vi "Get Points.vi"(11 "Task Base in":refnum<class "Task Base.lvclass">) -> (2 "Points":string[](array[string]), 3 "Task Base out":refnum<class "Task Base.lvclass">)   [LabVIEW 2023, in "Task Base.lvclass"]
uses:
  Task Base.lvclass
  Task Base.lvclass/Task Base.ctl
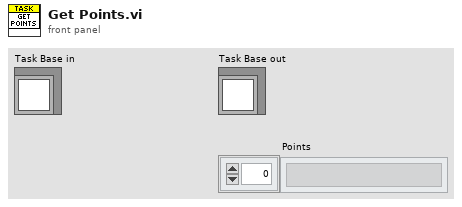
[diagram p1: front panel]
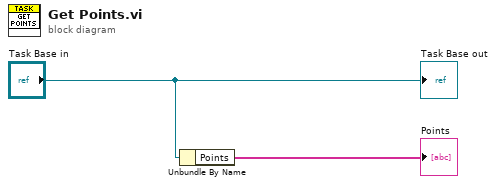
[diagram p0: block diagram]
diagram:
  n1 = Unbundle By Name("Task Base in") -> ("Points"=→"Points":string[])
  "Task Base out" <- "Task Base in"
